vi "labfinal.vi"() -> ()   [LabVIEW 2017]
doc: "This example demonstrates a simple PID position controller for a Quanser SRV-02 plant."
uses:
  <vilib>/Simulation/Scripting/Companion Diagram/SimConfigNode/SimParams.ctl
  <vilib>/Simulation/Scripting/Companion Diagram/SimConfigNode/_simSolvers.ctl
  <vilib>/Simulation/Implementation/Shared/SIMSCR Execution Mode.ctl
  <vilib>/Simulation/SignalArithmetic/Implementation/NILVSim Gain.llb/SIM Gain (scalar).vi
  <vilib>/Simulation/ContinuousLinear/Implementation/NILVSim Derivative.llb/SIM derivative (scalar).vi
  <vilib>/Simulation/Utility/Implementation/NILVSim Collector.llb/SIM Collector (scalar).vi
  <vilib>/Simulation/DataSources/Implementation/NILVSim Pulse Generator.llb/SIM Pulse Generator (scalar).vi
  <vilib>/Simulation/Nonlinear/Implementation/NILVSim Saturation.llb/SIM Saturation (scalar).vi
  <vilib>/Simulation/Utility/Implementation/SIM Halt.vi
  <vilib>/Simulation/Utility/Implementation/NILVSim Collector.llb/NILVSim Collector core (scalar).vi
  <vilib>/Simulation/Scripting/Companion Diagram/SimConfigNode/SimDog.xnode
  <vilib>/Quanser/Rapid Control Prototyping Toolkit/hardware/HIL Immediate IO/_TypeSpecific/CL HIL Read Encoder (Scalar).vi
  <vilib>/Quanser/Rapid Control Prototyping Toolkit/hardware/HIL Immediate IO/CL HIL Read.vi
  <vilib>/Quanser/Rapid Control Prototyping Toolkit/hardware/HIL Immediate IO/_TypeSpecific/CL HIL Write Analog (Scalar).vi
  <vilib>/Quanser/Rapid Control Prototyping Toolkit/hardware/HIL Immediate IO/CL HIL Write.vi
  <vilib>/Simulation/Implementation/XNodeFramework/SimXNode/SimX.xnode
  <vilib>/Simulation/Implementation/Shared/SIM Bundle Sim Info.vi
  <vilib>/Simulation/Implementation/Shared/SIM Unbundle Sim Info.vi
  <vilib>/Simulation/Implementation/Shared/NILVSim_FinalizeModel.vi
  <vilib>/Simulation/Implementation/Shared/NILVSim_GetModelError.vi
  <vilib>/Simulation/Utility/Implementation/NILVSim Get Time and IsAcceptedStep.vi
  <vilib>/Simulation/ContinuousLinear/Implementation/NILVSim Transfer Function.llb/SIM Transfer Function Collector (SISO).vi
  <vilib>/Simulation/ContinuousLinear/Implementation/NILVSim Transfer Function.llb/SIM Transfer Function Distributor (SISO).vi
  <vilib>/Simulation/Implementation/Shared/NILVSim_Manager.vi
  <vilib>/Simulation/Implementation/Shared/NILVSIM_BeginStep.vi
  <vilib>/Simulation/Implementation/Shared/NILVSim_Initialize.vi
  <vilib>/Simulation/Implementation/Shared/NILVSim_FinishedLate.vi
  <vilib>/Simulation/Param Hierarchy/Typedefs/SIMPH Param Control Actions.ctl
  <vilib>/Simulation/Implementation/Shared/NILVSim_ParamChanged.vi
  <vilib>/Platform/TimedLoop/XDataNode/timing_clust.ctl
  <vilib>/Platform/TimedLoop/XDataNode/wakeup.ctl
  <vilib>/Platform/TimedLoop/XDataNode/nitl_modes.ctl
  <vilib>/Utility/error.llb/Clear Errors.vi
  <vilib>/Simulation/Implementation/Shared/SIMSH Read Queue.vi
  <vilib>/Simulation/ContinuousLinear/Implementation/NILVSim Transfer Function.llb/SIM Transfer Function (SISO).vi
  <vilib>/Simulation/Implementation/Shared/NI_SIM_Implementation.lvlib
  <vilib>/Platform/TimedLoop/XDataNode/XDataNode.xnode
  <vilib>/Platform/TimedLoop/XDataNode/XDNodeRunTimeDep.lvlib
panel:
  in  "Stop Button":bool
  in  "Kd":dbl(knob)=0.15 scale=0.0..1.0
  in  "Kp":dbl(knob)=2.5 scale=1.0..4.0
  out "XY Graph":cluster{"Time":dbl[], "Signal":dbl[]}[](graph)
  out "Posição [rad]":T1(graph)
  out "encoder counts":i32=1029
  out "Error":errorcluster
  # "Controle PD"
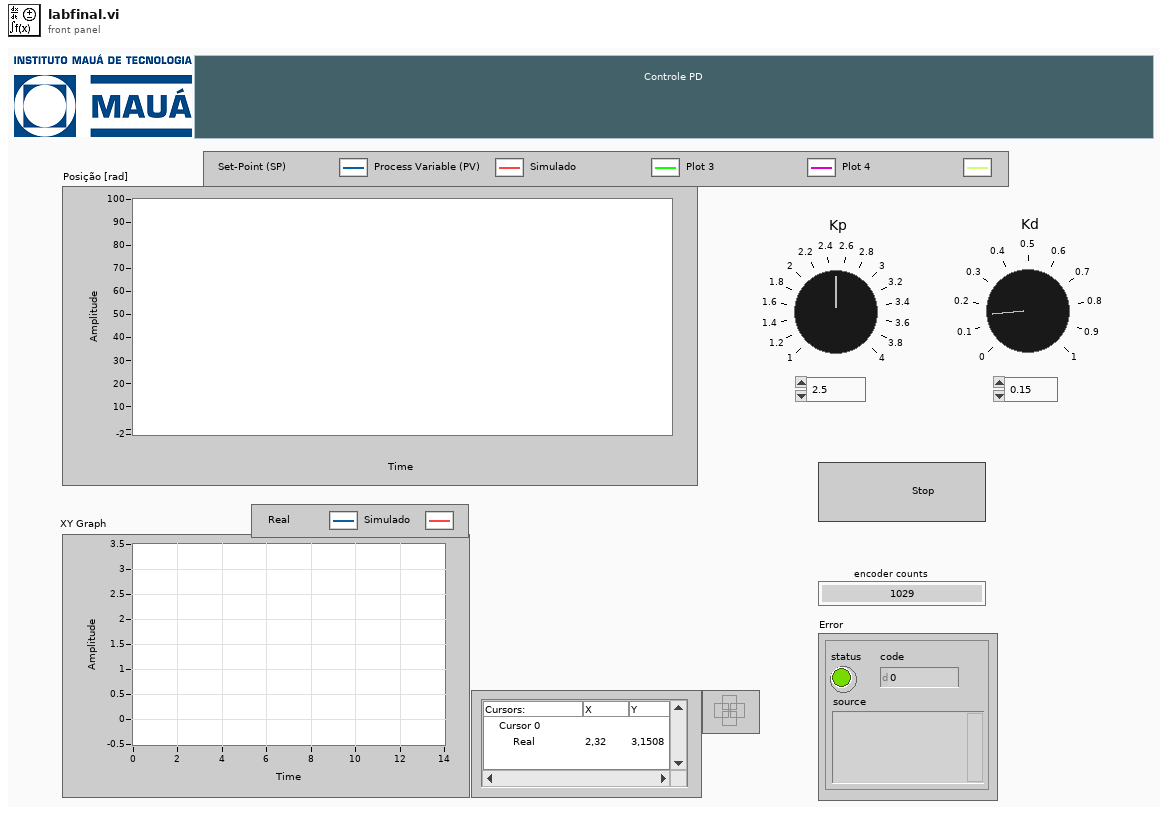
[diagram p1: front panel]
types:
  T1 = cluster{"output":dbl, "output":dbl, "output y(t)":dbl, "output":dbl, "output":dbl}
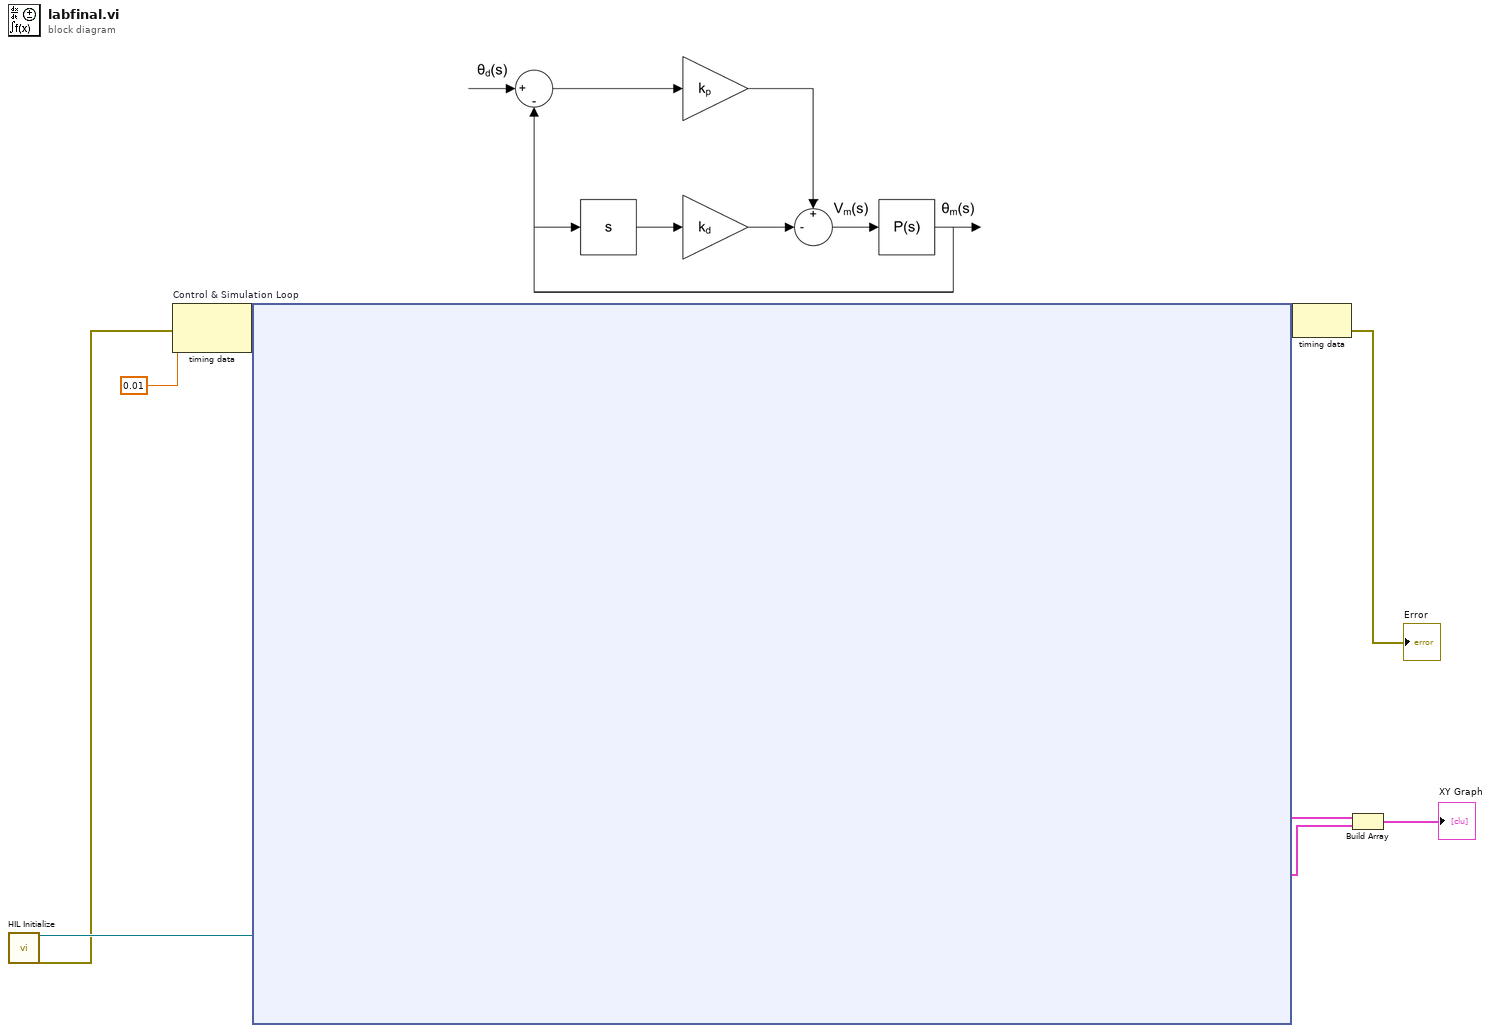
[diagram p0: block diagram]
diagram:
  n1 = call "HIL Initialize"() -> ("board out"=w7:refnum<class "HIL Board.lvclass">, "error out"=w4:errorcluster)  [unwired: 14 in]
  n2 = node-c288(w4, 0.01 ("Step Size (s)")) -> (w9:variant)
  n3 = node-c254 "Control & Simulation Loop"(w9, w7) -> (w8:variant, w3:cluster{"Time":dbl[], "Signal":dbl[]}, w1:cluster{"Time":dbl[], "Signal":dbl[]})
  n4 = node-c288(w8) -> (→"Error":errorcluster)
  n5 = Build Array "Build Array"(w3, w1) -> (→"XY Graph":cluster{"Time":dbl[], "Signal":dbl[]}[])
